vi "CPU_P_update_ZN.vi"(10 "value":u8 format="%02x", 11 "registers":T1={"A"=0, "X"=0, "Y"=0, "SP"=253, "PC"=0, "P"=36} {"P" format="%08b"; "PC" format="%04x"; "SP" format="%02x"; "Y" format="%02x"; "X" format="%02x"; "A" format="%02x"}) -> (3 "registers":T1={"A"=0, "X"=0, "Y"=0, "SP"=253, "PC"=0, "P"=36} {"P" format="%08b"; "PC" format="%04x"; "SP" format="%02x"; "Y" format="%02x"; "X" format="%02x"; "A" format="%02x"})   [LabVIEW 2018]
uses:
  CPU_registers.ctl
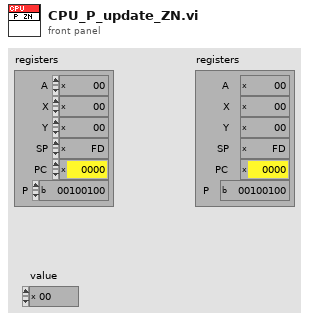
[diagram p1: front panel]
types:
  T1 = typedef "CPU_registers.ctl" = cluster{"A":u8, "X":u8, "Y":u8, "SP":u8, "PC":u16, "P":u8}
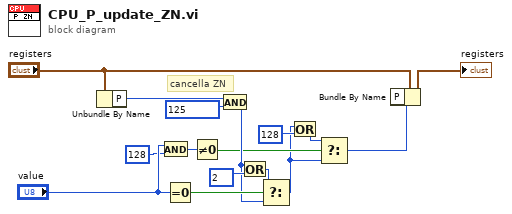
[diagram p0: block diagram]
diagram:
  # "cancella ZN"
  n1 = Unbundle By Name("registers") -> ("P"=w2:u8)
  n2 = And(x="value", y=u8 128) -> (x .and. y?=w11:u8)
  n3 = Equal To 0?(x="value") -> (x = 0?=w10:bool)
  n4 = Not Equal To 0?(x=w11) -> (x != 0?=w6:bool)
  n5 = And(x=w2, y=u8 125) -> (x .and. y?=w8:u8)
  n6 = Or(x=w8, y=u8 2) -> (x .or. y?=w7:u8)
  n7 = Select(t=w7, s=w10, f=w8) -> (s? t:f=w4:u8)
  n8 = Or(x=w4, y=u8 128) -> (x .or. y?=w3:u8)
  n9 = Select(t=w3, s=w6, f=w4) -> (s? t:f=w1:u8)
  n10 = Bundle By Name(cluster="registers", "P"=w1) -> (→"registers":T1)
